vi "MmsMain.vi"() -> ()   [LabVIEW 2017]
uses:
  <vilib>/NI/Software Watchdog/Pound/Pound.lvclass
  <vilib>/addons/InsightCM/Devices/Shared/Common/Trigger/Trigger.lvlib
  <vilib>/addons/TraceLogger/TraceLogger.lvlib
  <vilib>/addons/TimerProcess/TimerProcess.lvlib
  <vilib>/addons/WatchdogProcess/WatchdogProcess.lvlib
  <vilib>/addons/BlinkProcess/BlinkProcess.lvlib
  <vilib>/addons/InsightCM/Devices/Shared/Common/Controller/Controller.lvlib
  <vilib>/addons/InsightCM/Devices/Shared/Common/ServerComm/ServerComm.lvlib
  <vilib>/addons/InsightCM/Devices/Shared/Common/FileManager/FileManager.lvlib
  <vilib>/addons/InsightCM/Devices/Shared/Common/TracePointDisplay/TracePointDisplay.lvlib
  <vilib>/addons/InsightCM/Devices/Shared/Common/DataAccumulator/DataAccumulator.lvlib
  <vilib>/addons/InsightCM/Devices/Shared/Common/DeviceHealth/DeviceHealth.lvlib
  <vilib>/addons/InsightCM/Utilities/GlobalConfiguration/GlobalConfiguration.lvlib
  <vilib>/addons/InsightCM/Utilities/PropertyHelpers/PropertyHelpers.lvlib
  <vilib>/addons/InsightCM/Devices/Shared/Common/TrendAlarm/TrendAlarm.lvlib
  <vilib>/addons/InsightCM/Devices/Shared/Mcsa/McsaVirtualChannel/McsaVirtualChannel.lvlib
  <vilib>/addons/InsightCM/Devices/Shared/Mcsa/McsaAnalysisHighRate/McsaAnalysisHighRate.lvlib
  <vilib>/addons/InsightCM/Devices/Shared/Mcsa/McsaDataEventCreator/McsaDataEventCreator.lvlib
  <vilib>/addons/InsightCM/Devices/Shared/Mcsa/McsaAnalysisLowRate/McsaAnalysisLowRate.lvlib
  <vilib>/addons/InsightCM/Devices/Shared/Mcsa/McsaAnalysisLowUpdate/McsaAnalysisLowUpdate.lvlib
  <vilib>/addons/InsightCM/Devices/Shared/Mcsa/McsaTestPanel/McsaTestPanel.lvlib
  <vilib>/addons/InsightCM/Devices/Shared/Mcsa/McsaStartupAnalysis/McsaStartupAnalysis.lvlib
  <vilib>/addons/InsightCM/Devices/Shared/Mcsa/McsaFpgaAcquisition/McsaFpgaAcquisition.lvlib
  <vilib>/addons/InsightCM/Devices/Shared/Mcsa/McsaFpgaBitfileManager/McsaFpgaBitfileManager.lvlib
  <vilib>/addons/InsightCM/Devices/Shared/Mcsa/McsaOpState/McsaOpState.lvlib
  <vilib>/addons/InsightCM/Devices/Shared/Mcsa/McsaModbusMaster/McsaModbusMaster.lvlib
panel:
  out "debug":string
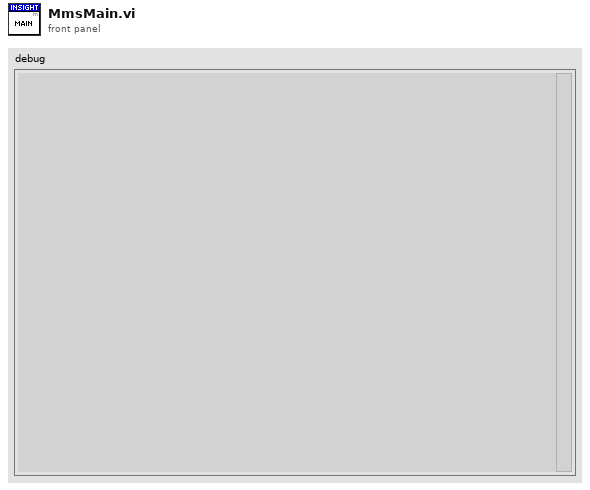
[diagram p1: front panel]
types:
  T1 = typedef "SectionKeyValues.ctl" = cluster{"Section":string, "KeyValues":T2[]}
  T2 = typedef "KeyValuePair.ctl" = cluster{"Key":string, "Value":string}
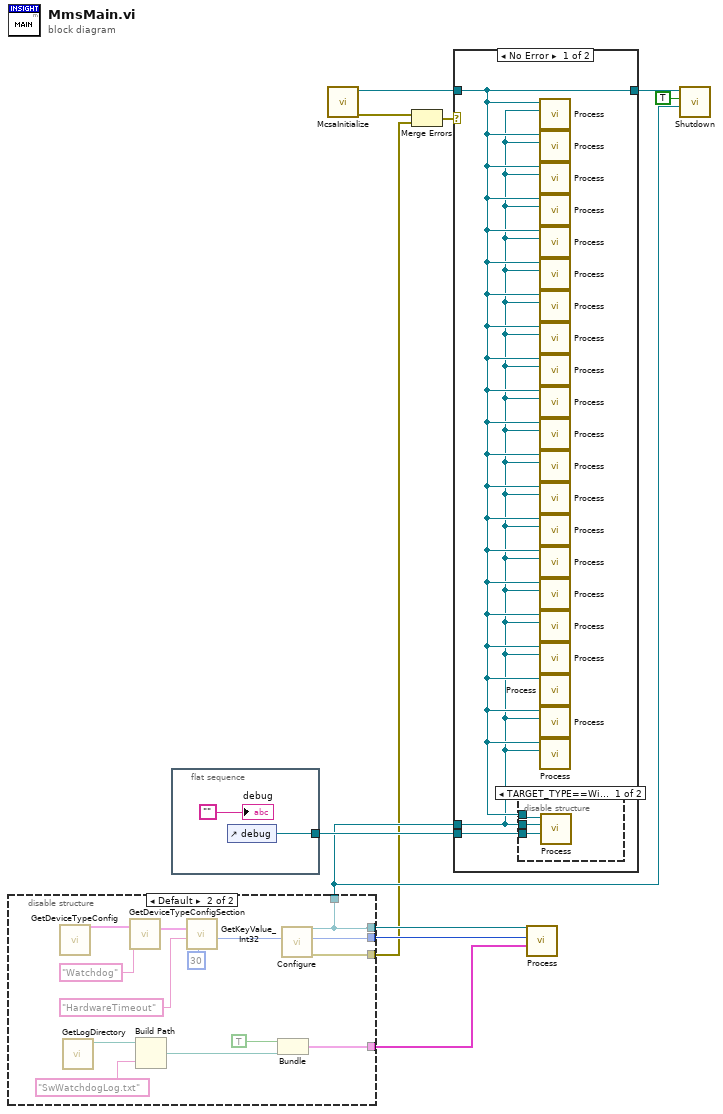
[diagram p0: block diagram]
diagram:
  n1 = disable-structure shown="Default" {
    disable-tunnel: [_ w25] -> w4
    disable-tunnel: [_ w25] -> w5
    disable-tunnel: [_ w24] -> w6
    disable-tunnel: [_ w14] -> w7
    disable-tunnel: [_ w12] -> w1
    frame condition #0 (active) {
    }
    frame condition #1 {
      n2 = call <vilib>:"GetDeviceTypeConfig.vi"() -> ("key values"=w19:T1[])  [unwired: 9 in, 2 out]
      n3 = call <vilib>:"GetLogDirectory.vi"() -> ("log dir"=w18:path)  [unwired: 10 in, 1 out]
      n4 = call <vilib>:"GetDeviceTypeConfigSection.vi"("key"="Watchdog", "key values"=w19) -> ("key value pairs out"=w22:T2[])  [unwired: 8 in, 1 out]
      n5 = Build Path(base path=w18, name or relative path="SwWatchdogLog.txt") -> (appended path=w16:path)
      n6 = call <vilib>:"GetKeyValue_Int32.vi"("default"=30, "key"="HardwareTimeout" ("Tag"), "key value pairs"=w22) -> ("value"=w13:i32)  [unwired: 6 in, 2 out]
      n7 = Bundle(TRUE, "appended path"=w16) -> (w14:cluster{bool, "appended path":path})  [unwired: 1 in]
      n8 = call <vilib>:"Configure.vi"("hw timeout (sec)"=w13) -> ("error out"=w12:errorcluster, "watchdogID out"=w24:u64, "Pound"=w25:refnum<class "Pound.lvclass">)  [unwired: 8 in]
    }
  }
  n9 = flat-sequence {
    tunnel: [w26] -> w10
    frame #0 {
      n10 = control-ref of="debug"() -> (w26:refnum<vi>)
      "debug" <- ""
    }
  }
  n11 = call <vilib>:"McsaInitialize.vi"() -> ("error out"=w3:errorcluster, "Qbus out"=w9:refnum<class "Qbus.lvclass">)  [unwired: 10 in]
  n12 = Merge Errors(w3, w1) -> (w2:errorcluster)
  n13 = case shown="No Error" w2 {
    tunnel: w9 -> [w29 w34]
    tunnel: [w29 w34] -> w11
    tunnel: w4 -> [w28 _]
    tunnel: w10 -> [w30 _]
    frame No Error {
      n14 = disable-structure shown="TARGET_TYPE==Windows" {
        disable-tunnel: w30 -> [w33 _]
        disable-tunnel: w29 -> [w32 _]
        disable-tunnel: w28 -> [w31 _]
        frame condition #0 (active) {
          n15 = call <vilib>:"Process.vi"("string refnum"=w33, "Pound in"=w31, "Qbus in"=w32) -> ()  [unwired: 8 in, 1 out]
        }
        frame condition #1 {
        }
      }
      n16 = call <vilib>:"Process.vi"("Pound in"=w28, "Qbus in"=w29) -> ()  [unwired: 9 in, 1 out]
      n17 = call <vilib>:"Process.vi"("Pound in"=w28, "Qbus in"=w29) -> ()  [unwired: 9 in, 1 out]
      n18 = call <vilib>:"Process.vi"("Pound in"=w28, "Qbus in"=w29) -> ()  [unwired: 9 in, 1 out]
      n19 = call <vilib>:"Process.vi"("Pound in"=w28, "Qbus in"=w29) -> ()  [unwired: 9 in, 1 out]
      n20 = call <vilib>:"Process.vi"("Pound in"=w28, "Qbus in"=w29) -> ()  [unwired: 9 in, 1 out]
      n21 = call <vilib>:"Process.vi"("Pound in"=w28, "Qbus in"=w29) -> ()  [unwired: 9 in, 1 out]
      n22 = call <vilib>:"Process.vi"("Pound in"=w28, "Qbus in"=w29) -> ()  [unwired: 9 in, 1 out]
      n23 = call <vilib>:"Process.vi"("pound in"=w28, "Qbus in"=w29) -> ()  [unwired: 9 in, 1 out]
      n24 = call <vilib>:"Process.vi"("Pound in"=w28, "Qbus in"=w29) -> ()  [unwired: 9 in, 1 out]
      n25 = call <vilib>:"Process.vi"("Pound in"=w28, "Qbus in"=w29) -> ()  [unwired: 9 in, 1 out]
      n26 = call <vilib>:"Process.vi"("Pound in"=w28, "Qbus in"=w29) -> ()  [unwired: 9 in, 1 out]
      n27 = call <vilib>:"Process.vi"("Pound in"=w28, "Qbus in"=w29) -> ()  [unwired: 9 in, 1 out]
      n28 = call <vilib>:"Process.vi"("Pound in"=w28, "Qbus in"=w29) -> ()  [unwired: 9 in, 1 out]
      n29 = call <vilib>:"Process.vi"("Pound in"=w28, "Qbus in"=w29) -> ()  [unwired: 9 in, 1 out]
      n30 = call <vilib>:"Process.vi"("Pound in"=w28, "Qbus in"=w29) -> ()  [unwired: 9 in, 1 out]
      n31 = call <vilib>:"Process.vi"("Pound in"=w28, "Qbus in"=w29) -> ()  [unwired: 9 in, 1 out]
      n32 = call <vilib>:"Process.vi"("Pound in"=w28, "Qbus in"=w29) -> ()  [unwired: 9 in, 1 out]
      n33 = call <vilib>:"Process.vi"("Pound in"=w28, "Qbus in"=w29) -> ()  [unwired: 9 in, 1 out]
      n34 = call <vilib>:"Process.vi"("qbus in"=w29) -> ()  [unwired: 10 in, 1 out]
      n35 = call <vilib>:"Process.vi"("Pound"=w28, "Qbus in"=w29) -> ()  [unwired: 9 in, 1 out]
      n36 = call <vilib>:"Process.vi"("pound in"=w28, "qbus in"=w29) -> ()  [unwired: 9 in, 1 out]
    }
    frame Error {
    }
  }
  n37 = call <vilib>:"Process.vi"("Logging"=w7, "watchdogID"=w6, "Pound"=w5) -> ()  [unwired: 6 in, 3 out]
  n38 = call <vilib>:"Shutdown.vi"("Pound"=w4, "restart system"=TRUE, "Qbus in"=w11) -> ()  [unwired: 8 in, 1 out]
